vi "UseClass.vi"() -> (3 "myClass.lvclass":refnum<class "myClass.lvclass">)   [LabVIEW 2010]
uses:
  myClass.lvclass
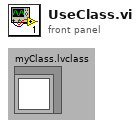
[diagram p1: front panel]
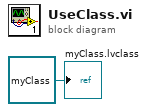
[diagram p0: block diagram]
diagram:
  "myClass.lvclass" <- refnum<class "myClass.lvclass"> refnum ("myClass.lvclass")
